vi "Close.vi"(8 "error in (no error)":errorcluster, 11 "ChromaPowerSupply in":refnum<class "ChromaPowerSupply.lvclass">) -> (0 "error out":errorcluster, 3 "ChromaPowerSupply out":refnum<class "ChromaPowerSupply.lvclass">)   [LabVIEW 2018, in "AcPwrPlugins.lvlib" / "ChromaPowerSupply.lvclass"]
doc: "This VI closes the reference to the instrument(s)."
uses:
  ChromaPowerSupply.lvclass
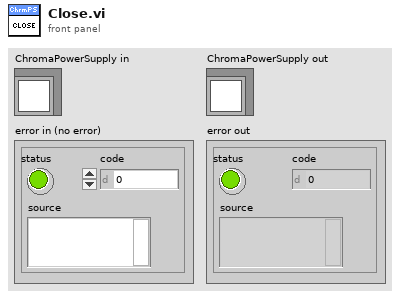
[diagram p1: front panel]
types:
  T1 = typedef "AcPwrPlugins.lvlib/ChromaPowerSupply.lvclass/Measurements.ctl" = cluster{"Handle":string, "Name":string, "Enabled":bool, "Measurement Value":dbl, "btnMeasFetch":bool, "ProtectionStatusString":string, "Measurement Type":enum16{"Voltage (V)", "Current (A)", "Power (W)"}}[]
  T2 = typedef "AcPwrPlugins.lvlib/ChromaPowerSupply.lvclass/Device(s)Settings.ctl" = cluster{"Phases":cluster{"Handle":string, "Instrument Options":string, "id query (T)":bool, "reset device (T)":bool, "Timing":cluster{"TimingOn":enum16{""}, "Hours":u32, "Minutes":u32, "Seconds":dbl, "CutoffVoltage":dbl}, "Connected":bool, "Output Mode":enum16{"Voltage (DC)", "Current (DC)"}, "Voltage":dbl, "Current":dbl, "Voltage Limit":dbl, "Current Limit":dbl}[], "MeasName":string}
  T3 = cluster{"Handle":string, "Instrument Options":string, "id query (T)":bool, "reset device (T)":bool, "Timing":cluster{"TimingOn":enum16{""}, "Hours":u32, "Minutes":u32, "Seconds":dbl, "CutoffVoltage":dbl}, "Connected":bool, "Output Mode":enum16{"Voltage (DC)", "Current (DC)"}, "Voltage":dbl, "Current":dbl, "Voltage Limit":dbl, "Current Limit":dbl}[]
  T4 = cluster{"Handle":string, "Instrument Options":string, "id query (T)":bool, "reset device (T)":bool, "Timing":cluster{"TimingOn":enum16{""}, "Hours":u32, "Minutes":u32, "Seconds":dbl, "CutoffVoltage":dbl}, "Connected":bool, "Output Mode":enum16{"Voltage (DC)", "Current (DC)"}, "Voltage":dbl, "Current":dbl, "Voltage Limit":dbl, "Current Limit":dbl}
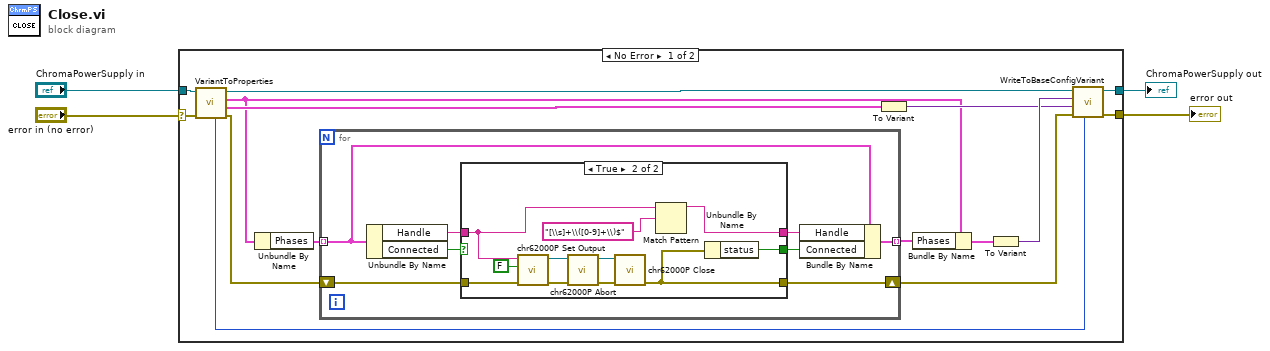
[diagram p0: block diagram]
diagram:
  n1 = case shown="No Error" "error in (no error)" {
    selector: "error in (no error)" -> [w18 w42]
    tunnel: [w10 w43] -> w2
    tunnel: "ChromaPowerSupply in" -> [w19 w43]
    tunnel: [w13 w42] -> w1
    frame No Error {
      n2 = call-dynamic "VariantToProperties.vi"("error in (no error)"=w18, "ChromaPowerSupply in"=w19) -> ("error out"=w16:errorcluster, "Measurements"=w9:T1, "Device Settings"=w6:T2, "ChromaPowerSupply out"=w11:refnum<class "ChromaPowerSupply.lvclass">, "Measurement Refresh Time (ms)"=w7:u32)  [unwired: 5 in]
      n3 = Unbundle By Name(w6) -> ("Phases"=w5:T3)
      n4 = for {
        tunnel: w5 -> [w27] mode=indexing
        shift-right: [w25] -> w14
        shift-left: w16 -> [w26]
        tunnel: [w24] -> w17 mode=indexing
        n5 = Unbundle By Name(w27) -> ("Handle"=w23:string, "Connected"=w20:bool)
        n6 = case shown="True" w20 {
          selector: w20 -> [w28 _]
          tunnel: w23 -> [w29 w33]
          tunnel: w26 -> [w30 w35]
          tunnel: [w30 w39] -> w25
          tunnel: [w29 w40] -> w22
          tunnel: [w28 w38] -> w21
          frame False {
          }
          frame True {
            n7 = call <instrlib>:"chr62000P Set Output.vi"("error in (no error)"=w35, "Output (Off)"=FALSE, "instrument handle"=w33) -> ("error out"=w34:errorcluster, "instrument handle out"=w32:refnum<k15>)  [unwired: 7 in]
            n8 = call <instrlib>:"chr62000P Abort.vi"("error in (no error)"=w34, "instrument handle"=w32) -> ("error out"=w37:errorcluster, "instrument handle out"=w36:refnum<k15>)  [unwired: 8 in]
            n9 = call <instrlib>:"chr62000P Close.vi"("error in (no error)"=w37, "instrument handle"=w36) -> ("error out"=w39:errorcluster)  [unwired: 9 in]
            n10 = Match Pattern(string=w33, regular expression="[\\s]+\\([0-9]+\\)$") -> (before substring=w40:string)  [unwired: 1 in, 3 out]
            n11 = Unbundle By Name(w39) -> ("status"=w38:bool)
          }
        }
        n12 = Bundle By Name(cluster=w27, "Handle"=w22, "Connected"=w21) -> (w24:T4)
      }
      n13 = To Variant(anything=w9) -> (Variant=w8:variant)
      n14 = Bundle By Name(cluster=w6, "Phases"=w17) -> (w15:T2)
      n15 = To Variant(anything=w15) -> (Variant=w12:variant)
      n16 = call-dynamic "WriteToBaseConfigVariant.vi"("Measurement Refresh Time (ms)"=w7, "error in (no error)"=w14, "Meas"=w8, "Config"=w12, "ChromaPowerSupply in"=w11) -> ("error out"=w13:errorcluster, "ChromaPowerSupply out"=w10:refnum<class "ChromaPowerSupply.lvclass">)  [unwired: 5 in]
    }
    frame Error {
    }
  }
  "error out" <- w1
  "ChromaPowerSupply out" <- w2
